vi "simulacion.vi"() -> ()   [LabVIEW 2018]
uses:
  <vilib>/Analysis/Matrix/Datatypes/RealMatrix.ctl
  <vilib>/Platform/TimedLoop/XDataNode/timing_clust.ctl
  <vilib>/Platform/TimedLoop/XDataNode/nitl_modes.ctl
  <vilib>/Platform/TimedLoop/XDataNode/wakeup.ctl
  <vilib>/Analysis/Matrix/Numeric/Conversions/Array To Matrix - RA.vi
  <vilib>/Analysis/Matrix/Numeric/Conversions/Array To Matrix - RA2.vi
  <vilib>/Analysis/Matrix/Numeric/Multiply/Multiply - RM,RM.vi
  <vilib>/Analysis/Matrix/Numeric/Add/Add - RM,RM.vi
  <vilib>/platform/TimedLoop/XDataNode/XDataNode.xnode
  <vilib>/Platform/TimedLoop/XDataNode/XDNodeRunTimeDep.lvlib
  <vilib>/Analysis/Matrix/NI_Matrix.lvlib
  <vilib>/Analysis/NI_AALPro.lvlib
panel:
  out "element":dbl
  out "A + B":T1
  out "Waveform Chart":dbl(graph)
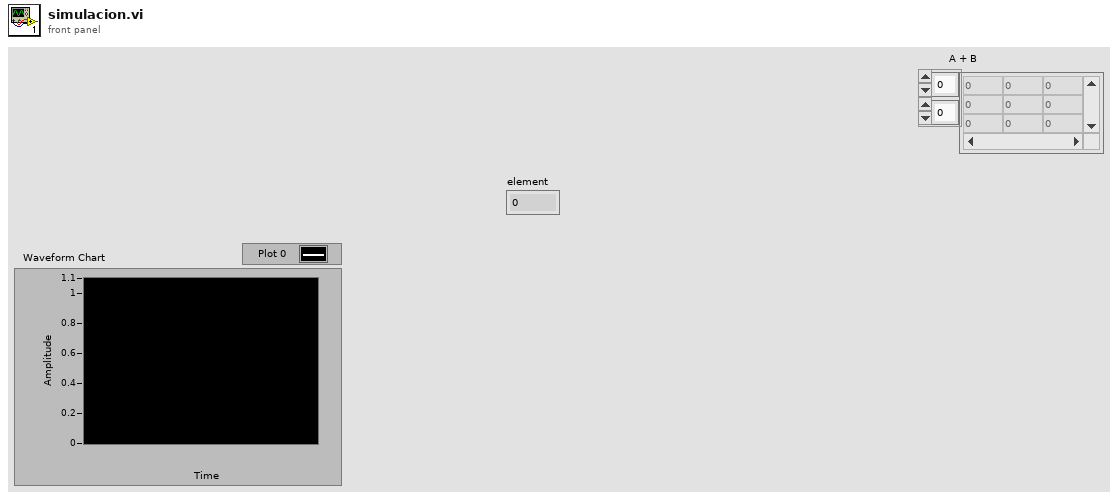
[diagram p1: front panel]
types:
  T1 = typedef "NI_Matrix.lvlib/RealMatrix.ctl" = dbl[][]
  T2 = typedef "XDNodeRunTimeDep.lvlib/timing_clust.ctl" = cluster{"Expected End [f-1]":u64, "Actual End [f-1]":u64, "Finished Late? [f-1]":bool, "Expected End [i-1]":u64, "Actual End [i-1]":u64, "Finished Late? [i-1]":bool, "Expected Start [i]":u64, "Actual Start [i]":u64, "Expected Start [f]":u64, "Actual Start [f]":u64, "Source Name":string, "Structure Name":string, "Period":i64, "Deadline":i64, "Offset":i64, "Start":i64, "Priority":i32, "Timeout":i32, "Mode":T3, "Wakeup Reason":T4, "Error":errorcluster, "Source Type":string, "Secondary Source Type":string, "Global End Time":u64, "Global Start Time":u64, "Frame Duration":u64, "Iteration Duration":u64, "Assigned CPU":i32, "I/O Scan Engine Mode":u32}
  T3 = typedef "XDNodeRunTimeDep.lvlib/nitl_modes.ctl" = enum32{"No Change", "Process missed periods, maintain original phase", "Discard missed periods, maintain original phase", "Process missed periods, ignore original phase", "Discard missed periods, ignore original phase"}
  T4 = typedef "XDNodeRunTimeDep.lvlib/wakeup.ctl" = enum32{"Normal", "Aborted", "Asynchronous wakeup", "Timing source error", "Timed loop error", "Timeout"}
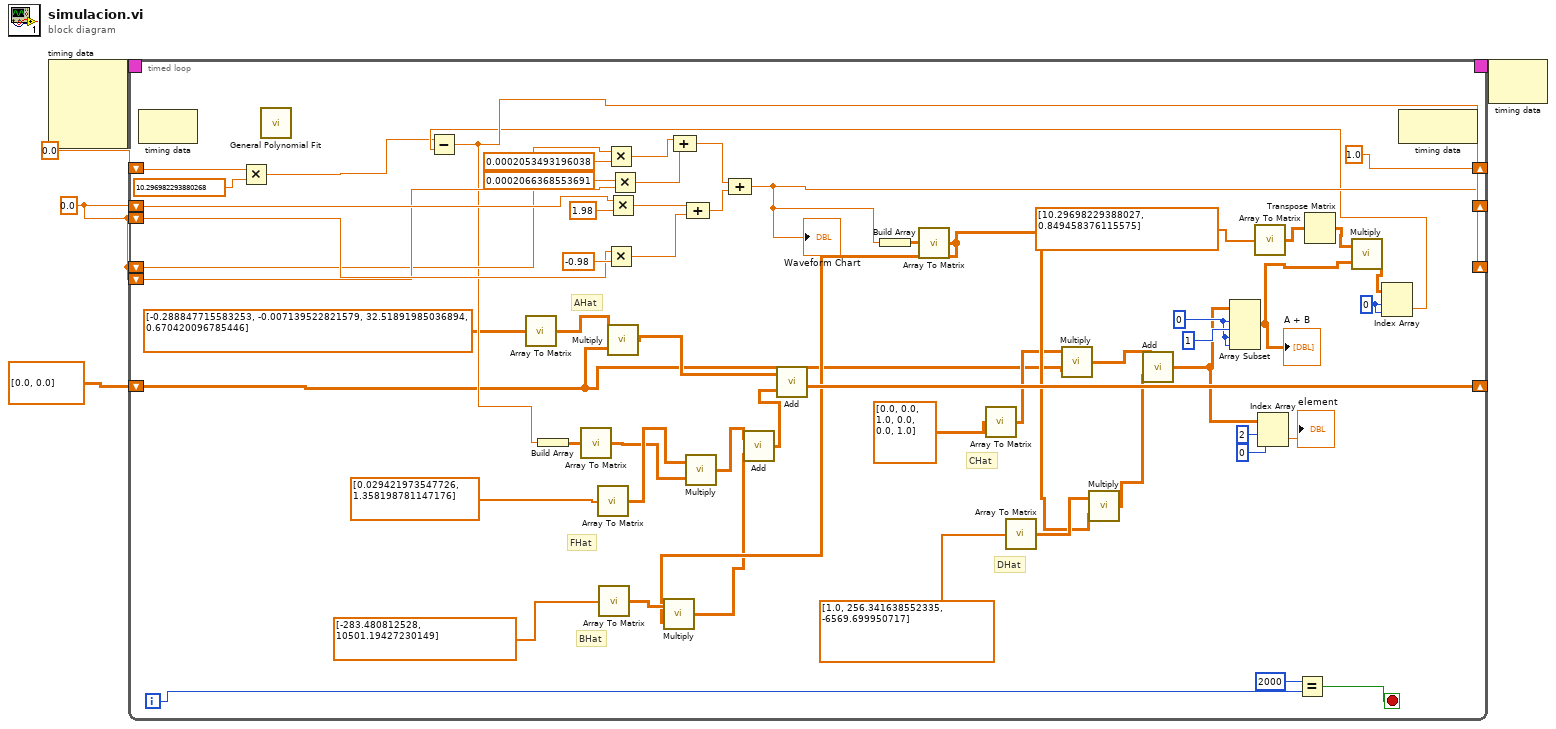
[diagram p0: block diagram]
diagram:
  w1 = 0.0
  n1 = node-c288() -> (w5:T2)  [unwired: 4 in]
  n2 = timed-loop {
    timing: w5 -> [_]
    timing-out: [_] -> w4
    shift-right: [w39] -> _
    shift-left: w1 -> [w59]
    shift-left: w1 -> [w58]
    shift-right: [1.0] -> _
    shift-left: 0.0 -> [w12]
    shift-right: [w42] -> _
    shift-left: T1 [[0.0], [0.0]] ("A + B") -> [w22]
    shift-right: [w40] -> _
    shift-left: w1 -> [w43]
    shift-left: w1 -> [w44]
    i -> [w16]
    stop <- w14 stop-if-true
    w45 = 0 ("index (row)")
    w47 = 0 ("row 1")
    # "DHat"
    # "CHat"
    # "FHat"
    # "AHat"
    # "BHat"
    n3 = node-c288() -> ()  [unwired: 1 in, 1 out]
    n4 = Multiply ("Multiply.vi")(x=w12, y=10.296982293880268) -> (x*y=w10:dbl)
    n5 = call <vilib>:"General Polynomial Fit.vi"() -> ()  [unwired: 12 in, 4 out]
    n6 = call-poly <vilib>:"Array To Matrix.vi"("Real 2D Array"=dbl[][] [[-0.288847715583253, -0.007139522821579], [32.51891985036894, 0.670420096785446]] ("element")) -> ("Real Matrix"=w32:T1)
    n7 = call-poly <vilib>:"Array To Matrix.vi"("Real 1D Array"=dbl[] [0.029421973547726, 1.358198781147176] ("element")) -> ("Real Matrix (Column Vector)"=w30:T1)
    n8 = call-poly <vilib>:"Array To Matrix.vi"("Real 1D Array"=dbl[] [-283.480812528, 10501.19427230149] ("element")) -> ("Real Matrix (Column Vector)"=w27:T1)
    n9 = Multiply(x=w43, y=0.0002053493196038) -> (x*y=w55:dbl)
    n10 = Multiply(x=w58, y=-0.98) -> (x*y=w62:dbl)
    n11 = Multiply(x=w59, y=1.98) -> (x*y=w63:dbl)
    n12 = call-poly <vilib>:"Multiply.vi"("Real Matrix B"=w22, "Real Matrix A"=w32) -> ("A * B"=w31:T1)
    n13 = Multiply(x=0.0002066368553691 ("y"), y=w44) -> (x*y=w54:dbl)
    n14 = Compound Arithmetic op=ADD(w55, w54) -> (w53:dbl)
    n15 = Compound Arithmetic op=ADD(w63, w62) -> (w52:dbl)
    n16 = Compound Arithmetic op=ADD(w53, w52) -> (w39:dbl)
    "Waveform Chart" <- w39
    n17 = Build Array(w39) -> (w49:T1)
    n18 = call-poly <vilib>:"Array To Matrix.vi"("Real 2D Array"=w49) -> ("Real Matrix"=w26:T1)
    n19 = call-poly <vilib>:"Multiply.vi"("Real Matrix B"=w26, "Real Matrix A"=w27) -> ("A * B"=w25:T1)
    n20 = call-poly <vilib>:"Array To Matrix.vi"("Real 2D Array"=dbl[][] [[0.0, 0.0], [1.0, 0.0], [0.0, 1.0]]) -> ("Real Matrix"=w23:T1)
    n21 = call-poly <vilib>:"Array To Matrix.vi"("Real 1D Array"=dbl[] [1.0, 256.341638552335, -6569.699950717] ("element")) -> ("Real Matrix (Column Vector)"=w33:T1)
    n22 = call-poly <vilib>:"Multiply.vi"("Real Matrix B"=w22, "Real Matrix A"=w23) -> ("A * B"=w21:T1)
    n23 = call-poly <vilib>:"Multiply.vi"("Real Matrix B"=w26, "Real Matrix A"=w33) -> ("A * B"=w24:T1)
    n24 = call-poly <vilib>:"Add.vi"("Real Matrix B"=w24, "Real Matrix A"=w21) -> ("A + B"=w9:T1)
    n25 = Array Subset(array=w9, index (row)=w47, length (row)=1 ("row N"), index (col)=w47, length (col)=w47) -> (w19:T1)
    "A + B" <- w19
    n26 = call-poly <vilib>:"Array To Matrix.vi"("Real 1D Array"=dbl[] [10.29698229388027, 0.849458376115575] ("element")) -> ("Real Matrix (Column Vector)"=w46:T1)
    n27 = Index Array(array=w9, index (row)=2, index (col)=0) -> (element=→"element":dbl)
    n28 = Equal?(x=2000, y=w16) -> (x = y?=w14:bool)
    n29 = Transpose Matrix(1:w46) -> (0:w20:T1)
    n30 = call-poly <vilib>:"Multiply.vi"("Real Matrix B"=w19, "Real Matrix A"=w20) -> ("A * B"=w18:T1)
    n31 = Index Array(array=w18, index (row)=w45, index (col)=w45) -> (element=w13:dbl)
    n32 = Subtract(x=w10, y=w13) -> (x-y=w40:dbl)
    n33 = Build Array(w40) -> (w50:T1)
    n34 = call-poly <vilib>:"Array To Matrix.vi"("Real 2D Array"=w50) -> ("Real Matrix"=w29:T1)
    n35 = call-poly <vilib>:"Multiply.vi"("Real Matrix B"=w29, "Real Matrix A"=w30) -> ("A * B"=w28:T1)
    n36 = call-poly <vilib>:"Add.vi"("Real Matrix B"=w25, "Real Matrix A"=w28) -> ("A + B"=w41:T1)
    n37 = call-poly <vilib>:"Add.vi"("Real Matrix B"=w41, "Real Matrix A"=w31) -> ("A + B"=w42:T1)
    n38 = node-c288() -> ()  [unwired: 1 in, 1 out]
  }
  n39 = node-c288(w4) -> ()  [unwired: 1 out]
